vi "CursorDataGraphMove_vis.vi"(4 "timedelays":dbl[](array[numeric]), 5 "wavelengths":dbl[](array[numeric]), 6 "Data":sgl[][](array[numeric]), 7 "References":T1) -> ()   [LabVIEW 2018, in "Control-Client.lvclass"]
uses:
  Control-Client.lvclass
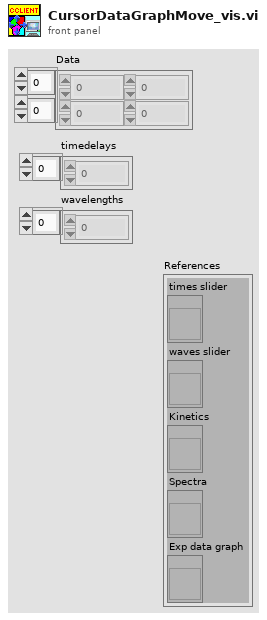
[diagram p1: front panel]
types:
  T1 = cluster{"times slider":refnum<vi>, "waves slider":refnum<vi>, "Kinetics":refnum<vi>, "Spectra":refnum<vi>, "Exp data graph":refnum<vi>}
  T2 = cluster{"Max Y pixel":i32, "Min Y pixel":i32, "Max X pixel":i32, "Min X pixel":i32}
  T3 = cluster{"From Time, pix":i32, "To Time, pix":i32, "From Wave, pix":i32, "To Wave, pix":i32}
  T4 = cluster{"From Time":dbl, "To Time":dbl, "From Wave":dbl, "To Wave":dbl}
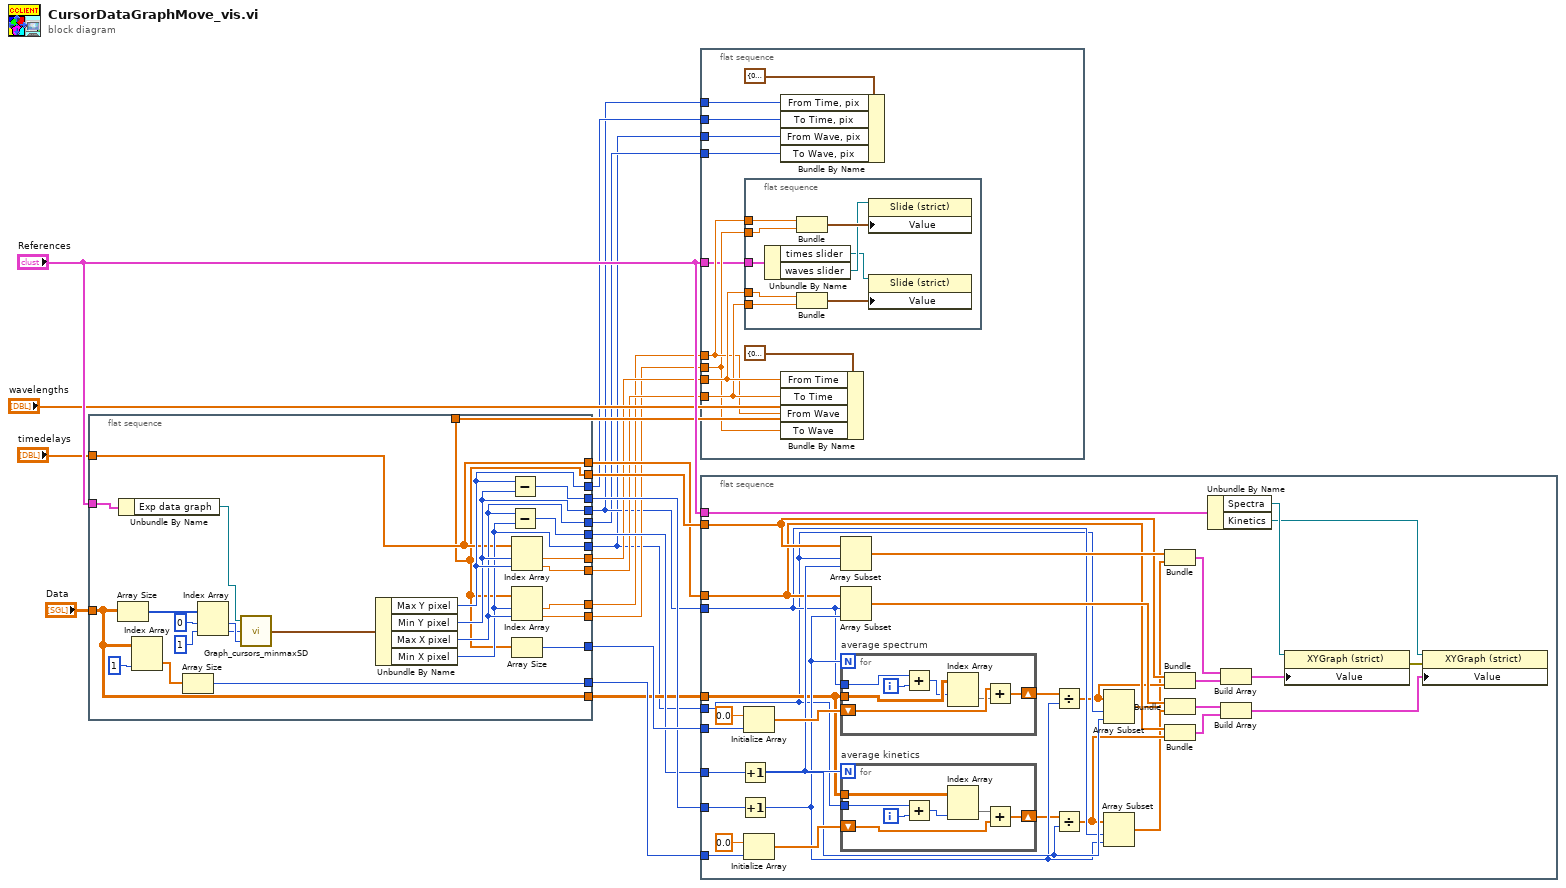
[diagram p0: block diagram]
diagram:
  n1 = flat-sequence {
    tunnel: [w43] -> w15
    tunnel: [w42] -> w14
    tunnel: [w40] -> w13
    tunnel: [w39] -> w12
    tunnel: [w20] -> w11
    tunnel: [w21] -> w10
    tunnel: [w24] -> w9
    tunnel: [w37] -> w8
    tunnel: [w36] -> w7
    tunnel: [w35] -> w6
    tunnel: [w34] -> w5
    tunnel: [w33] -> w4
    tunnel: [w32] -> w3
    tunnel: [w31] -> w2
    tunnel: [w30] -> w1
    tunnel: "Data" -> [w24]
    tunnel: "References" -> [w23]
    tunnel: "timedelays" -> [w21]
    tunnel: "wavelengths" -> [w20]
    frame #0 {
      n2 = Array Size(array=w24) -> (size(s)=w29:i32[])
      n3 = Unbundle By Name(w23) -> ("Exp data graph"=w22:refnum<vi>)
      n4 = Index Array(array=w24, index (col)=1 ("disabled index (col)")) -> (element=w44:sgl[])  [unwired: 1 in]
      n5 = Array Size(array=w44) -> (size(s)=w43:i32)
      n6 = Index Array(array=w29, index #1=0 ("index"), index #2=1 ("index")) -> (element #1=w26:i32, element #2=w25:i32)
      n7 = call "Graph_cursors_minmaxSD.vi"("Max Y pixel"=w26, "Max X pixel"=w25, "GRAPH EXPERIMENTAL DATA"=w22) -> ("max/min XY pixels"=w41:T2)
      n8 = Unbundle By Name(w41) -> ("Max Y pixel"=w33:i32, "Min Y pixel"=w32:i32, "Max X pixel"=w31:i32, "Min X pixel"=w30:i32)
      n9 = Subtract(x=w33, y=w32) -> (x-y=w40:i32)
      n10 = Subtract(x=w31, y=w30) -> (x-y=w39:i32)
      n11 = Index Array(array=w21, index #1=w32, index #2=w33) -> (element #1=w37:dbl, element #2=w36:dbl)
      n12 = Index Array(array=w20, index #1=w30, index #2=w31) -> (element #1=w35:dbl, element #2=w34:dbl)
      n13 = Array Size(array=w20) -> (size(s)=w42:i32)
    }
  }
  n14 = flat-sequence {
    tunnel: w8 -> [w55]
    tunnel: w7 -> [w54]
    tunnel: w6 -> [w53]
    tunnel: w5 -> [w52]
    tunnel: w4 -> [w51]
    tunnel: w3 -> [w50]
    tunnel: w2 -> [w49]
    tunnel: w1 -> [w48]
    tunnel: "References" -> [w47]
    frame #0 {
      n15 = flat-sequence {
        tunnel: w55 -> [w64]
        tunnel: w54 -> [w63]
        tunnel: w53 -> [w62]
        tunnel: w52 -> [w61]
        tunnel: w47 -> [w60]
        frame #0 {
          n16 = Unbundle By Name(w60) -> ("times slider"=w56:refnum<vi>, "waves slider"=w57:refnum<vi>)
          n17 = Bundle("Numeric"=w62, "Numeric"=w61) -> (w59:cluster{"Numeric":dbl, "Numeric":dbl})  [unwired: 1 in]
          n18 = Bundle("delay"=w64, "delay"=w63) -> (w58:cluster{"delay":dbl, "delay":dbl})  [unwired: 1 in]
          n19 = property class="Slide (strict)"(reference=w57, "Value"=w59) -> ()  [unwired: 1 in, 2 out]
          n20 = property class="Slide (strict)"(reference=w56, "Value"=w58) -> ()  [unwired: 1 in, 2 out]
        }
      }
      n21 = Bundle By Name(cluster=T3 {"From Time, pix"=0, "To Time, pix"=0, "From Wave, pix"=0, "To Wave, pix"=0} ("output cluster"), "From Time, pix"=w50, "To Time, pix"=w51, "From Wave, pix"=w48, "To Wave, pix"=w49) -> ()  [unwired: 1 out]
      n22 = Bundle By Name(cluster=T4 {"From Time"=0.0, "To Time"=0.0, "From Wave"=0.0, "To Wave"=0.0} ("output cluster"), "From Time"=w55, "To Time"=w54, "From Wave"=w53, "To Wave"=w52) -> ()  [unwired: 1 out]
    }
  }
  n23 = flat-sequence {
    tunnel: w15 -> [w95]
    tunnel: w14 -> [w94]
    tunnel: w13 -> [w89]
    tunnel: w12 -> [w88]
    tunnel: w11 -> [w85]
    tunnel: w10 -> [w84]
    tunnel: w9 -> [w83]
    tunnel: w3 -> [w82]
    tunnel: w1 -> [w81]
    tunnel: "References" -> [w70]
    frame #0 {
      n24 = Increment(x=w88) -> (x+1=w91:i32)
      n25 = Increment(x=w89) -> (x+1=w86:i32)
      n26 = Initialize Array(0.0 ("element"), w94) -> (w92:dbl[])
      n27 = Initialize Array(0.0 ("element"), w95) -> (w97:dbl[])
      n28 = Array Subset(array=w85, index=w81, length=w91) -> (w87:dbl[])
      n29 = Array Subset(array=w84, index=w82, length=w86) -> (w90:dbl[])
      n30 = for "average spectrum" {
        N: w86 -> [_]
        shift-right: [w104] -> w77
        shift-left: w92 -> [w101]
        tunnel: w82 -> [w102]
        tunnel: w83 -> [w100]
        i -> [w103]
        n31 = Add(x=w102, y=w103) -> (x+y=w99:i32)
        n32 = Index Array(array=w100, index (row)=w99) -> (element=w98:sgl[])  [unwired: 1 in]
        n33 = Add(x=w101, y=w98) -> (x+y=w104:dbl[])
      }
      n34 = for "average kinetics" {
        N: w91 -> [_]
        tunnel: w83 -> [w111]
        tunnel: w81 -> [w109]
        shift-right: [w105] -> w80
        shift-left: w97 -> [w106]
        i -> [w110]
        n35 = Add(x=w109, y=w110) -> (x+y=w108:i32)
        n36 = Index Array(array=w111, index (col)=w108) -> (element=w107:sgl[])  [unwired: 1 in]
        n37 = Add(x=w107, y=w106) -> (x+y=w105:dbl[])
      }
      n38 = Divide(x=w77, y=w86) -> (x/y=w76:dbl[])
      n39 = Divide(x=w80, y=w91) -> (x/y=w79:dbl[])
      n40 = Array Subset(array=w76, index=w81, length=w91) -> (w75:dbl[])
      n41 = Array Subset(array=w79, index=w82, length=w86) -> (w78:dbl[])
      n42 = Bundle(w87, w75) -> (w74:cluster{dbl[], dbl[]})  [unwired: 1 in]
      n43 = Bundle("wavelengths"=w85, w76) -> (w73:cluster{"wavelengths":dbl[], dbl[]})  [unwired: 1 in]
      n44 = Bundle(w90, w78) -> (w72:cluster{dbl[], dbl[]})  [unwired: 1 in]
      n45 = Bundle("timedelays"=w84, w79) -> (w71:cluster{"timedelays":dbl[], dbl[]})  [unwired: 1 in]
      n46 = Unbundle By Name(w70) -> ("Spectra"=w69:refnum<vi>, "Kinetics"=w67:refnum<vi>)
      n47 = Build Array(w74, w73) -> (w66:cluster{"wavelengths":dbl[], dbl[]}[])
      n48 = Build Array(w72, w71) -> (w65:cluster{"timedelays":dbl[], dbl[]}[])
      n49 = property class="XYGraph (strict)"(reference=w69, "Value"=w66) -> (error out=w68:errorcluster)  [unwired: 1 in, 1 out]
      n50 = property class="XYGraph (strict)"(reference=w67, error in=w68, "Value"=w65) -> ()  [unwired: 2 out]
    }
  }
